vi "Voronoi_Boundary Edges Area.vi"(9 "P 3":dbl[](array[numeric]), 10 "P 2":dbl[](array[numeric]), 11 "P 1":dbl[](array[numeric])) -> (3 "area":dbl)   [LabVIEW 2020, in "NI_AAL_Geometry.lvlib"]
uses:
  <vilib>/Analysis/NI_AAL_Geometry.lvlib
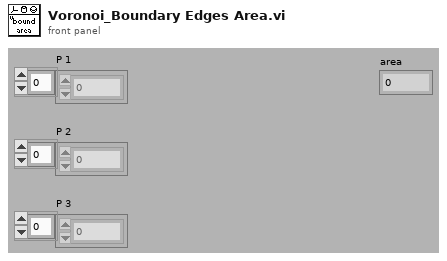
[diagram p1: front panel]
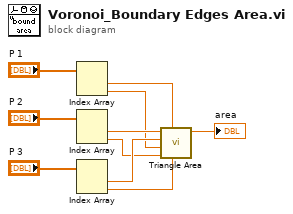
[diagram p0: block diagram]
diagram:
  n1 = Index Array(array="P 1") -> (element #1=w7:dbl, element #2=w3:dbl)  [unwired: 2 in]
  n2 = Index Array(array="P 2") -> (element #1=w6:dbl, element #2=w2:dbl)  [unwired: 2 in]
  n3 = Index Array(array="P 3") -> (element #1=w5:dbl, element #2=w4:dbl)  [unwired: 2 in]
  n4 = call <vilib>:"Triangle Area.vi"("y 3"=w4, "x 1"=w7, "y 2"=w2, "y 1"=w3, "x 3"=w5, "x 2"=w6) -> ("area"=→"area":dbl)  [unwired: 5 out]
